vi "suasGroundStation.vi"() -> ()   [LabVIEW 2011]
panel:
  out "AverageTimePerMessage":dbl
  out "Alive":bool
  in  "Rebalance":bool
  in  "streamBool":bool
  out "size(s)":i32
  out "# elements in queue":i32
  out "Completed Images":u16[](array[numeric])
  out "OutputImages":T1(array[cluster])
  out "queue out":refnum<queue>
  out "port":u16
  out "address":u32
  in  "stop":bool
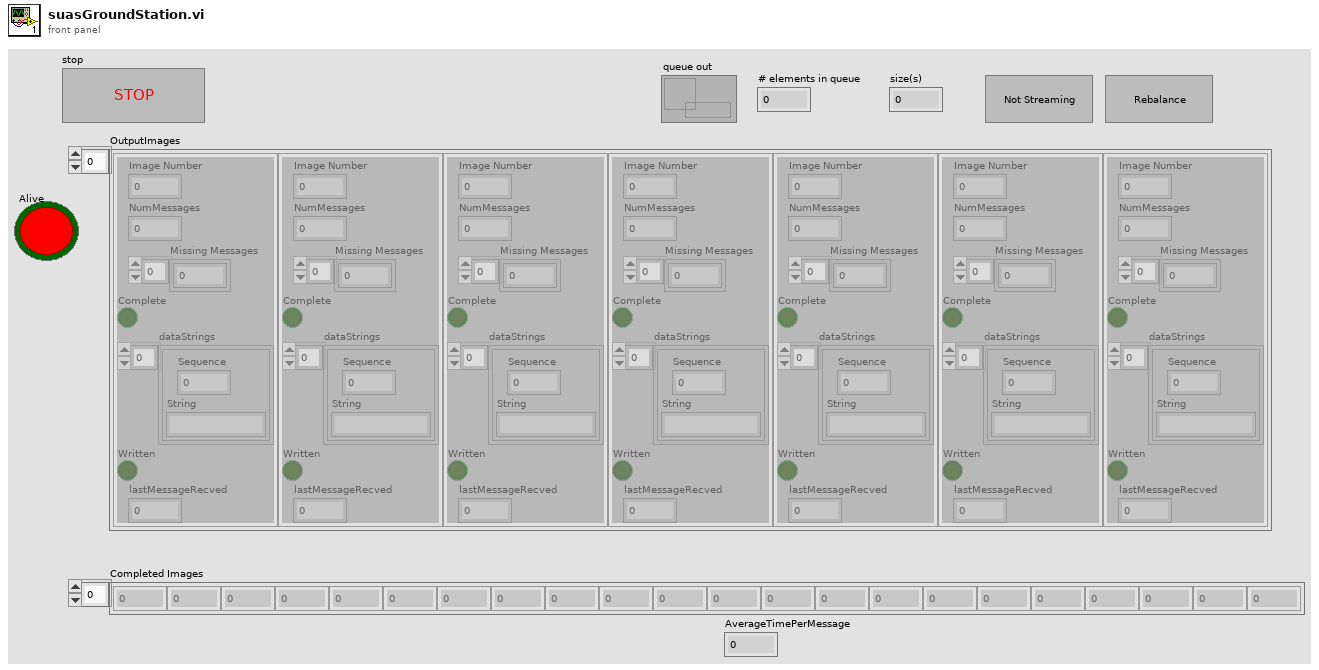
[diagram p1: front panel]
types:
  T1 = cluster{"Image Number":u16, "NumMessages":u16, "Missing Messages":u16[], "Complete":bool, "dataStrings":cluster{"Sequence":u16, "String":string}[], "Written":bool, "lastMessageRecved":u32}[]
  T2 = cluster{"Image Number":i32, "millisecond timer value":u32}[]
  T3 = cluster{"Image Number":i32, "millisecond timer value":u32}
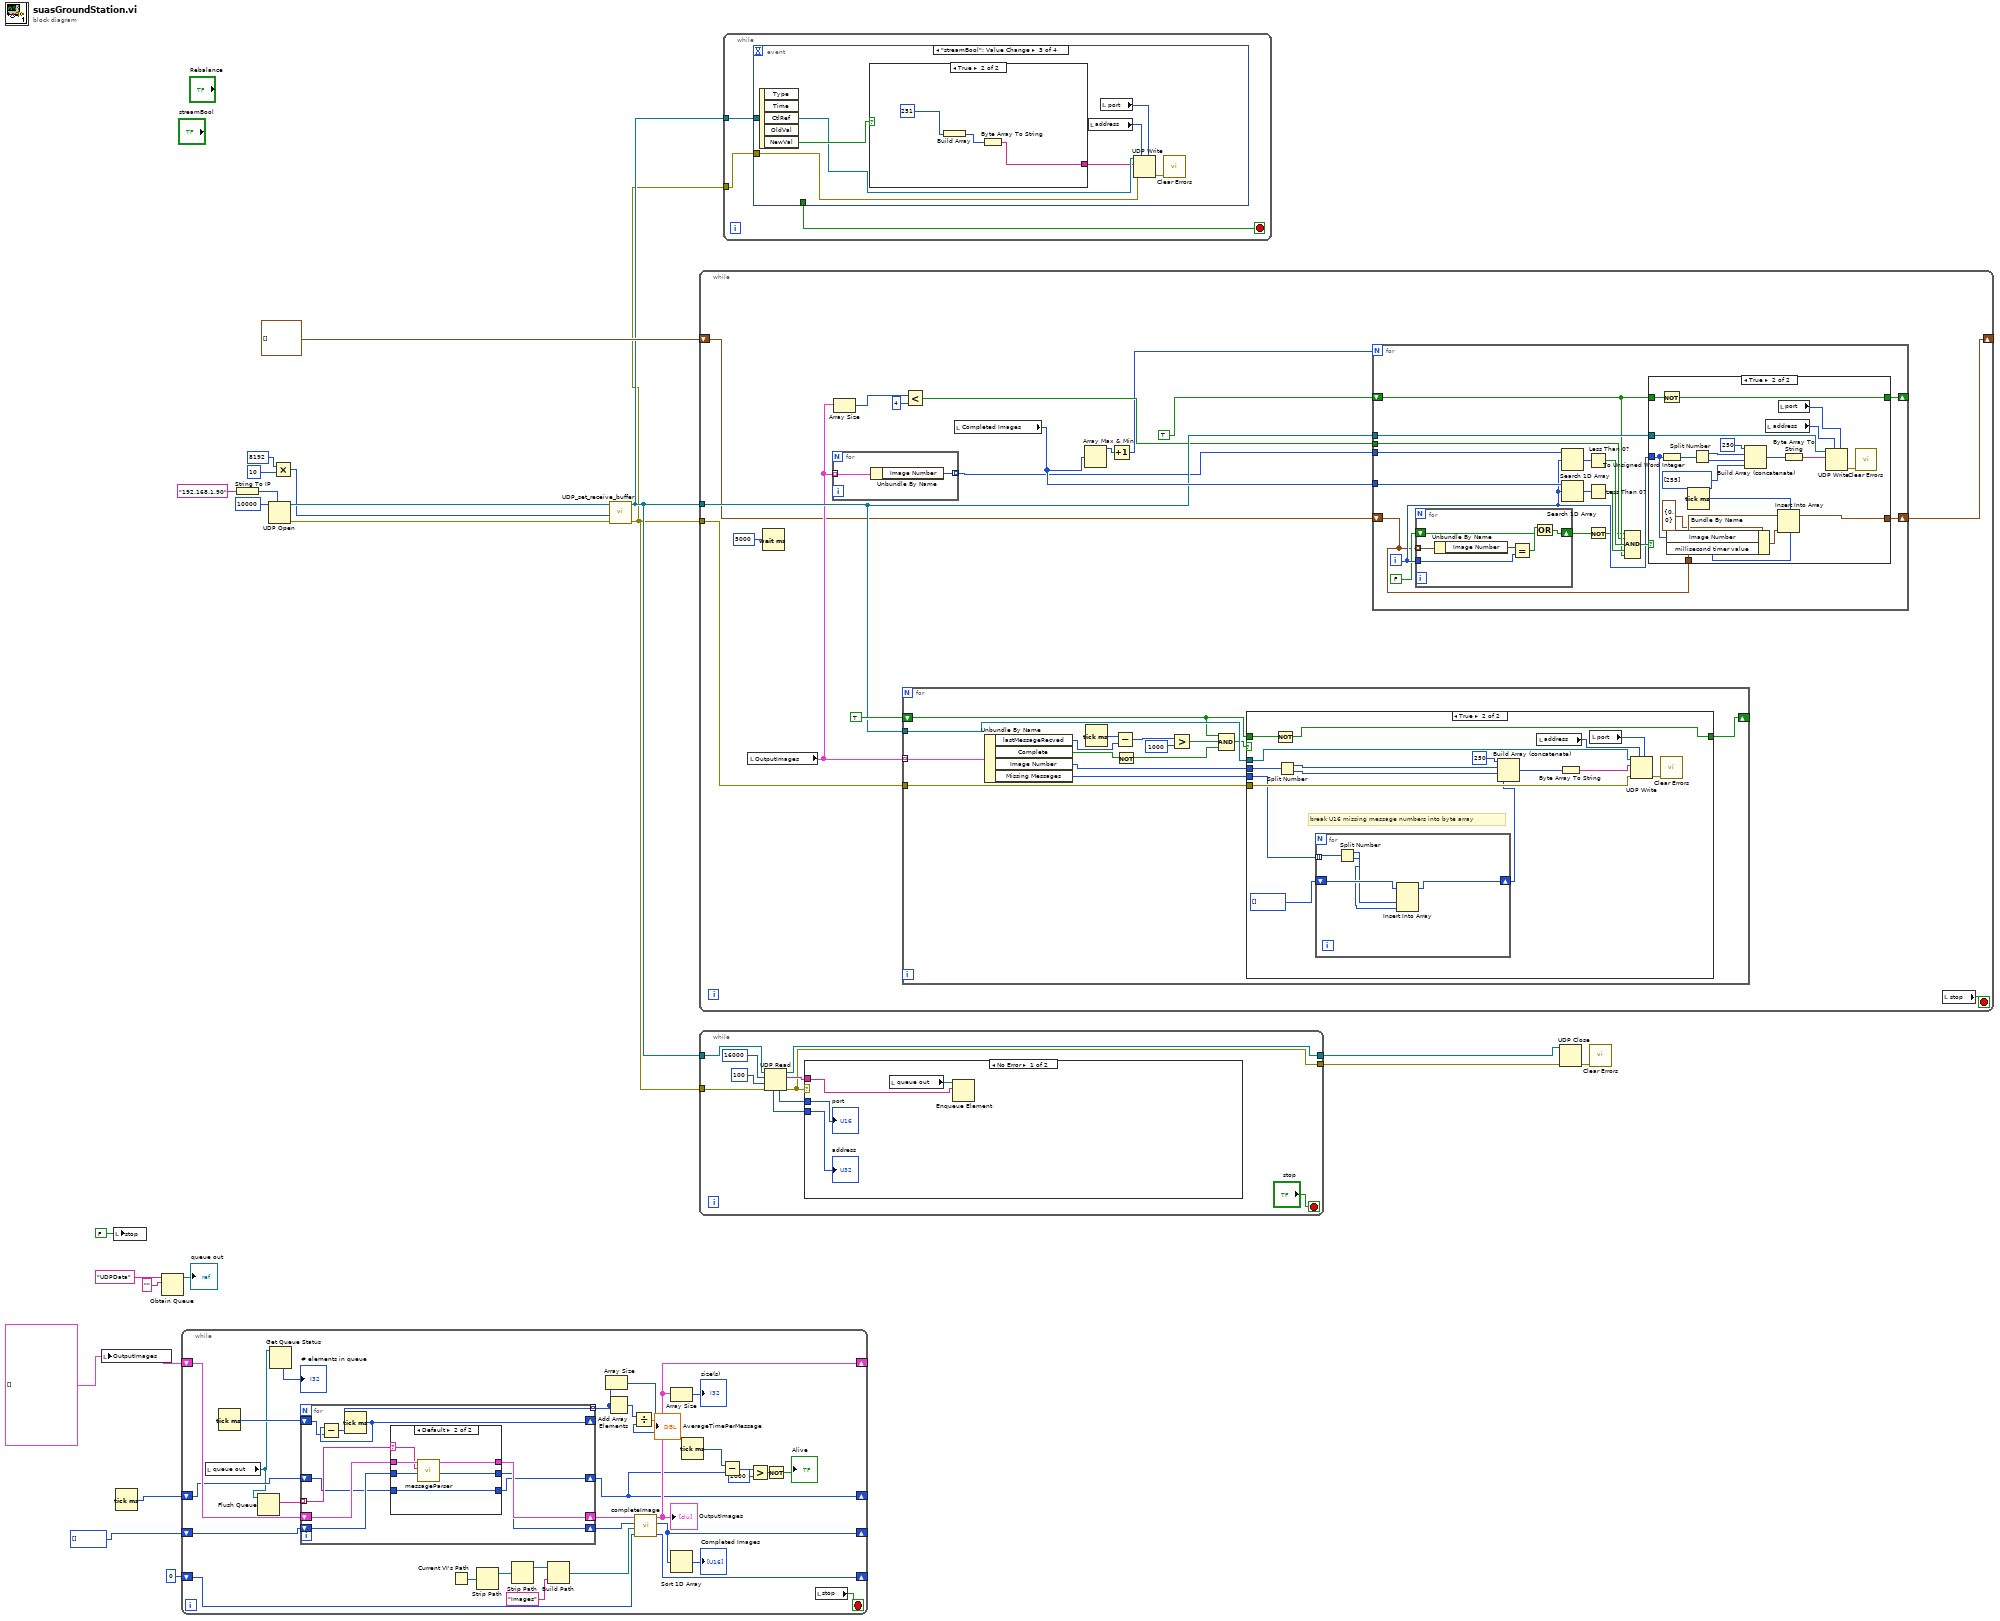
[diagram p0: block diagram]
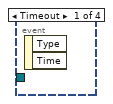
[diagram p2: hidden frame]
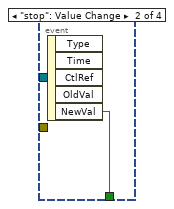
[diagram p3: hidden frame]
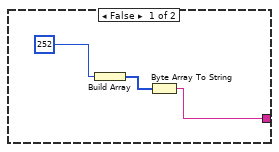
[diagram p4: hidden frame]
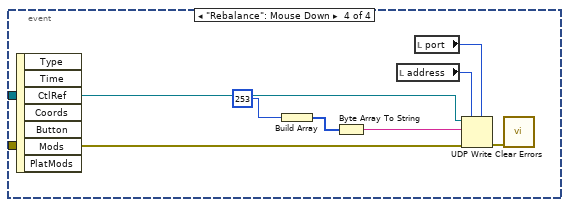
[diagram p5: hidden frame]
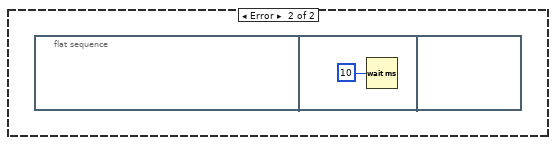
[diagram p8: hidden frame]
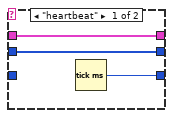
[diagram p9: hidden frame]
diagram:
  w7 = T1 [] ("OutputImages 2")
  n1 = local write "OutputImages"(w7) -> ()
  n2 = local write "stop"(FALSE ("stop")) -> ()
  n3 = Tick Count (ms)() -> (millisecond timer value=w1:u32)
  n4 = Obtain Queue(name (unnamed)="UDPData", element data type="") -> (queue out=→"queue out":refnum<queue>)  [unwired: 3 in, 2 out]
  n5 = while {
    shift-right: [w47] -> _
    shift-left: w7 -> [w52]
    shift-right: [w50] -> _
    shift-left: u16[] [] ("Array 2") -> [w51]
    shift-right: [w42] -> _
    shift-left: 0 ("Numeric 2") -> [w43]
    shift-right: [w39] -> _
    shift-left: w1 -> [w41]
    stop <- w53 stop-if-true
    n6 = local read "queue out"() -> (w29:refnum<queue>)
    n7 = Tick Count (ms)() -> (millisecond timer value=w34:u32)
    n8 = Flush Queue(queue=w29) -> (remaining elements=w28:string[])  [unwired: 1 in, 2 out]
    n9 = Get Queue Status(queue=w29) -> (# elements in queue=→"# elements in queue":i32)  [unwired: 2 in, 7 out]
    n10 = for {
      shift-right: [w62] -> w45
      shift-left: w52 -> [w63]
      shift-right: [w60] -> w44
      shift-left: w51 -> [w61]
      tunnel: w28 -> [w59] mode=indexing
      shift-right: [w58] -> w39
      shift-left: w41 -> [w57]
      shift-right: [w56] -> _
      shift-left: w34 -> [w55]
      tunnel: [w54] -> w33 mode=indexing
      n11 = Tick Count (ms)() -> (millisecond timer value=w56:u32)
      n12 = Subtract(x=w56, y=w55) -> (x-y=w54:u32)
      n13 = case shown="Default" w59 {
        selector: w59 -> [_ w68]
        tunnel: w63 -> [w66 w72]
        tunnel: [w66 w71] -> w62
        tunnel: w61 -> [w65 w70]
        tunnel: [w65 w69] -> w60
        tunnel: [w64 w67] -> w58
        tunnel: w57 -> [_ w67]
        frame "heartbeat" {
          n14 = Tick Count (ms)() -> (millisecond timer value=w64:u32)
        }
        frame Default {
          n15 = call "messageParser.vi"("Completed Images In"=w70, "Input"=w68, "Input Images"=w72) -> ("Completed Images Out"=w69:u16[], "OutputImages"=w71:T1)  [unwired: 7 in]
        }
      }
    }
    n16 = Current VI's Path() -> (path=w27:path)
    n17 = Strip Path(path=w27) -> (stripped path=w26:path)  [unwired: 1 out]
    n18 = Strip Path(path=w26) -> (stripped path=w25:path)  [unwired: 1 out]
    n19 = Build Path(base path=w25, name or relative path="Images") -> (appended path=w23:path)
    n20 = Array Size(array=w33) -> (size(s)=w31:i32)
    n21 = Add Array Elements(numeric array=w33) -> (sum=w32:u32)
    n22 = Divide(x=w32, y=w31) -> (x/y=→"AverageTimePerMessage":dbl)
    n23 = call "completeImage.vi"("Numeric"=w43, "file (use dialog)"=w23, "Array"=w44, "InputImages"=w45) -> ("Numeric 2"=w42:i32, "Array 2"=w50:u16[], "OutputImages"=w47:T1)  [unwired: 5 in]
    "OutputImages" <- w47
    n24 = Array Size(array=w47) -> (size(s)=→"size(s)":i32)
    n25 = Sort 1D Array(array=w50) -> (sorted array=→"Completed Images":u16[])
    n26 = Tick Count (ms)() -> (millisecond timer value=w40:u32)
    n27 = Subtract(x=w40, y=w39) -> (x-y=w38:u32)
    n28 = Greater?(x=w38, y=u32 2000) -> (0:w36:bool)
    n29 = Not(x=w36) -> (.not. x?=→"Alive":bool)
    n30 = local read "stop"() -> (w53:bool)
  }
  n31 = String To IP(1:"192.168.1.90" ("name")) -> (0:w21:u32)
  n32 = UDP Open(7:w21, 11:u16 10000 ("port")) -> (port=w12:refnum<k16>, 0:w11:errorcluster)  [unwired: 3 in, 1 out]
  n33 = Multiply(x=u32 8192 ("Receive Buffer Size"), y=u32 10) -> (x*y=w8:u32)
  n34 = call "UDP_set_receive_buffer.vi"("error in (no error)"=w11, "Receive Buffer Size"=w8, "connection ID"=w12) -> ("error out"=w3:errorcluster, "connection ID out"=w4:refnum<k16>)  [unwired: 6 in]
  n35 = while {
    tunnel: w4 -> [w83]
    tunnel: w3 -> [w87]
    shift-right: [w73] -> _
    shift-left: T2 [] -> [w74]
    stop <- w88 stop-if-true
    n36 = local read "OutputImages"() -> (w81:T1)
    n37 = Wait (ms)(milliseconds to wait=u32 5000) -> ()  [unwired: 1 out]
    n38 = for {
      tunnel: w81 -> [w134] mode=indexing
      tunnel: [w133] -> w82 mode=indexing
      n39 = Unbundle By Name(w134) -> ("Image Number"=w133:u16)
    }
    n40 = Array Size(array=w81) -> (size(s)=w80:i32)
    n41 = for {
      tunnel: w83 -> [w149]
      tunnel: w87 -> [w148]
      tunnel: w81 -> [w145] mode=indexing
      shift-right: [w142] -> _
      shift-left: TRUE -> [w136]
      n42 = Unbundle By Name(w145) -> ("lastMessageRecved"=w139:u32, "Complete"=w144:bool, "Image Number"=w147:u16, "Missing Messages"=w146:u16[])
      n43 = Tick Count (ms)() -> (millisecond timer value=w140:u32)
      n44 = Subtract(x=w140, y=w139) -> (x-y=w138:u32)
      n45 = Not(x=w144) -> (.not. x?=w141:bool)
      n46 = Greater?(x=w138, y=u32 1000) -> (0:w135:bool)
      n47 = Compound Arithmetic op=AND(w136, w135, w141) -> (w143:bool)
      n48 = case shown="True" w143 {
        tunnel: w149 -> [_ w166]
        tunnel: w148 -> [_ w165]
        tunnel: w147 -> [_ w156]
        tunnel: w146 -> [_ w152]
        tunnel: w136 -> [w150 w155]
        tunnel: [w150 w154] -> w142
        frame False {
        }
        frame True {
          # "break U16 missing message numbers into byte array"
          n49 = Not(x=w155) -> (.not. x?=w154:bool)
          n50 = Split Number(x=w156) -> (hi(x)=w159:u8, lo(x)=w161:u8)
          n51 = for {
            tunnel: w152 -> [w171] mode=indexing
            shift-right: [w167] -> w151
            shift-left: u8[] [] -> [w170]
            n52 = Split Number(x=w171) -> (hi(x)=w169:u8, lo(x)=w168:u8)
            n53 = Insert Into Array(array=w170, new element #1=w169, new element #2=w168) -> (w167:u8[])  [unwired: 1 in]
          }
          n54 = Build Array (concatenate)(u8 250, w159, w161, w151) -> (w160:u8[])
          n55 = local read "address"() -> (w163:u32)
          n56 = Byte Array To String(unsigned byte array=w160) -> (string=w158:string)
          n57 = local read "port"() -> (w164:u16)
          n58 = UDP Write(address=w163, port or service name=w164, connection ID=w166, data in=w158, 8:w165) -> (error out=w157:errorcluster)  [unwired: 1 in, 1 out]
          n59 = call <vilib>:"Clear Errors.vi"("error in (no error)"=w157) -> ()  [unwired: 6 in, 1 out]
        }
      }
    }
    n60 = Less?(x=w80, y=4) -> (x < y?=w78:bool)
    n61 = local read "Completed Images"() -> (w84:u16[])
    n62 = Array Max & Min(array=w84) -> (max value=w77:u16)  [unwired: 3 out]
    n63 = Increment(x=w77) -> (x+1=w76:u16)
    n64 = for {
      N: w76 -> [_]
      tunnel: w84 -> [w105]
      tunnel: w82 -> [w104]
      tunnel: w83 -> [w98]
      shift-right: [w97] -> _
      shift-left: TRUE -> [w96]
      tunnel: w78 -> [w95]
      shift-right: [w89] -> w73
      shift-left: w74 -> [w90]
      i -> [w94]
      n65 = for {
        tunnel: w90 -> [w111] mode=indexing
        tunnel: w94 -> [w109]
        shift-right: [w106] -> w92
        shift-left: FALSE -> [w107]
        n66 = Unbundle By Name(w111) -> ("Image Number"=w110:i32)
        n67 = Equal?(x=w110, y=w109) -> (x = y?=w108:bool)
        n68 = Or(x=w108, y=w107) -> (x .or. y?=w106:bool)
      }
      n69 = Search 1D Array(1D array=w104, element=w94) -> (index of element=w102:i32)  [unwired: 1 in]
      n70 = Search 1D Array(1D array=w105, element=w94) -> (index of element=w103:i32)  [unwired: 1 in]
      n71 = Less Than 0?(x=w102) -> (x < 0?=w101:bool)
      n72 = Less Than 0?(x=w103) -> (x < 0?=w100:bool)
      n73 = Not(x=w92) -> (.not. x?=w91:bool)
      n74 = Compound Arithmetic op=AND(w91, w95, w101, w100, w96) -> (w99:bool)
      n75 = case shown="True" w99 {
        tunnel: w98 -> [_ w122]
        tunnel: w94 -> [_ w116]
        tunnel: w96 -> [w113 w121]
        tunnel: [w113 w120] -> w97
        tunnel: w90 -> [w112 w119]
        tunnel: [w112 w118] -> w89
        frame False {
        }
        frame True {
          n76 = Not(x=w121) -> (.not. x?=w120:bool)
          n77 = To Unsigned Word Integer(number=w116) -> (unsigned 16bit integer=w123:u16)
          n78 = Tick Count (ms)() -> (millisecond timer value=w115:u32)
          n79 = Bundle By Name(cluster=T3 {"Image Number"=0, "millisecond timer value"=0} ("new element/subarray"), "Image Number"=w116, "millisecond timer value"=w115) -> (w114:T3)
          n80 = Split Number(x=w123) -> (hi(x)=w127:u8, lo(x)=w129:u8)
          n81 = Build Array (concatenate)(u8 250, w127, w129, u8[] [255] ("array")) -> (w128:u8[])
          n82 = local read "address"() -> (w131:u32)
          n83 = Insert Into Array(array=w119, new element=w114) -> (w118:T2)  [unwired: 1 in]
          n84 = local read "port"() -> (w132:u16)
          n85 = Byte Array To String(unsigned byte array=w128) -> (string=w126:string)
          n86 = UDP Write(address=w131, port or service name=w132, connection ID=w122, data in=w126) -> (error out=w125:errorcluster)  [unwired: 2 in, 1 out]
          n87 = call <vilib>:"Clear Errors.vi"("error in (no error)"=w125) -> ()  [unwired: 6 in, 1 out]
        }
      }
    }
    n88 = local read "stop"() -> (w88:bool)
  }
  n89 = while {
    tunnel: w4 -> [w180]
    tunnel: w3 -> [w179]
    tunnel: [w178] -> w19
    tunnel: [w174] -> w18
    stop <- "stop" stop-if-true
    n90 = UDP Read(connection ID=w180, max size (548)=16000, timeout ms (25000)=100, 8:w179) -> (data out=w176:string, error out=w174:errorcluster, 3:w178:refnum<k16>, 4:w172:u16, 6:w173:u32)
    n91 = case shown="No Error" w174 {
      tunnel: w176 -> [w183 _]
      tunnel: w173 -> [w185 _]
      tunnel: w172 -> [w184 _]
      frame No Error {
        n92 = local read "queue out"() -> (w182:refnum<queue>)
        n93 = Enqueue Element(queue=w182, element=w183) -> ()  [unwired: 2 in, 3 out]
        "address" <- w185
        "port" <- w184
      }
      frame Error {
        n94 = flat-sequence {
          frame #0 {
          }
          frame #1 {
            n95 = Wait (ms)(milliseconds to wait=u32 10) -> ()  [unwired: 1 out]
          }
          frame #2 {
          }
        }
      }
    }
  }
  n96 = while {
    tunnel: w4 -> [w188]
    tunnel: w3 -> [w187]
    stop <- w189 stop-if-true
    n97 = event shown="[2] \"streamBool\": Value Change" {
      selector: _ -> [_ _ _ _]
      dyn-events: _ -> [_ _ _ _]
      timeout: _ -> [_ _ _ _]
      tunnel: [_ w190 _ _] -> w189
      tunnel: w188 -> [_ _ w195 w205]
      tunnel: w187 -> [_ _ w194 w204]
      event Timeout {
        n98 = event-data() -> ()  [unwired: 1 in, 2 out]
      }
      event "stop": Value Change {
        n99 = event-data() -> ("NewVal"=w190:bool)  [unwired: 1 in, 4 out]
      }
      event "streamBool": Value Change {
        n100 = event-data() -> ("NewVal"=w197:bool)  [unwired: 1 in, 4 out]
        n101 = case shown="True" w197 {
          tunnel: [w198 w201] -> w193
          frame False {
            n102 = Build Array(u8 252) -> (w200:u8[])
            n103 = Byte Array To String(unsigned byte array=w200) -> (string=w198:string)
          }
          frame True {
            n104 = Build Array(u8 251) -> (w203:u8[])
            n105 = Byte Array To String(unsigned byte array=w203) -> (string=w201:string)
          }
        }
        n106 = local read "address"() -> (w192:u32)
        n107 = local read "port"() -> (w191:u16)
        n108 = UDP Write(address=w192, port or service name=w191, connection ID=w195, data in=w193, 8:w194) -> (error out=w196:errorcluster)  [unwired: 1 in, 1 out]
        n109 = call <vilib>:"Clear Errors.vi"("error in (no error)"=w196) -> ()  [unwired: 6 in, 1 out]
      }
      event "Rebalance": Mouse Down {
        n110 = event-data() -> ()  [unwired: 1 in, 7 out]
        n111 = Build Array(u8 253) -> (w208:u8[])
        n112 = Byte Array To String(unsigned byte array=w208) -> (string=w206:string)
        n113 = local read "address"() -> (w210:u32)
        n114 = local read "port"() -> (w209:u16)
        n115 = UDP Write(address=w210, port or service name=w209, connection ID=w205, data in=w206, 8:w204) -> (error out=w211:errorcluster)  [unwired: 1 in, 1 out]
        n116 = call <vilib>:"Clear Errors.vi"("error in (no error)"=w211) -> ()  [unwired: 6 in, 1 out]
      }
    }
  }
  n117 = UDP Close(connection ID=w19, 8:w18) -> (error out=w17:errorcluster)  [unwired: 1 out]
  n118 = call <vilib>:"Clear Errors.vi"("error in (no error)"=w17) -> ()  [unwired: 6 in, 1 out]
